vi "LimelightDistanceEstimator.vi"(1 "TargetHeight":dbl, 2 "Ty":dbl) -> (0 "Distance Estimate":dbl)   [LabVIEW 2018]
doc: "Takes in Target center pixel Y value (ty) and outputs the estimated distance of the target from the camera. This requires knowing the Angle the camera makes with the horizontal, camera height from ground, and target height from ground. Target height from ground is a required input."
panel:
  in  "CameraHeight":dbl
  in  "CameraAngle":dbl
  # "FIXED CAMERA ANGLE DISTANCE ESTIMATOR"
  # "This will be how far below the horizontal the camera views, since we've put it super high up and angled it down. \nPlease, just keep this number positive, in degrees"
  # "This is in inches. Measure from the floor, to the center of the lense."
  # "This is in inches. Measure from the floor, to the middle of the target (line connecting midpoints of angled tape inner edge)"
  # "Outputted Distance Estimate"
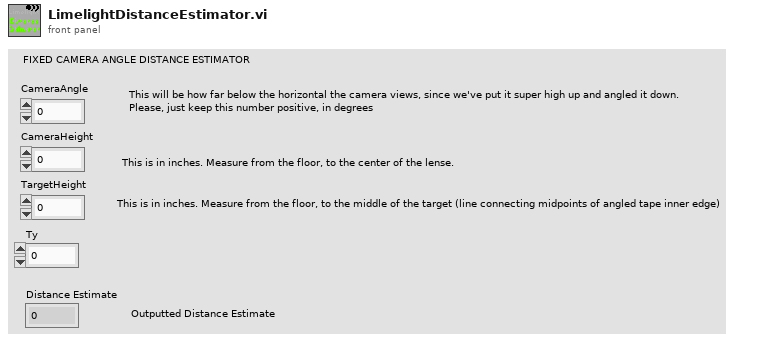
[diagram p1: front panel]
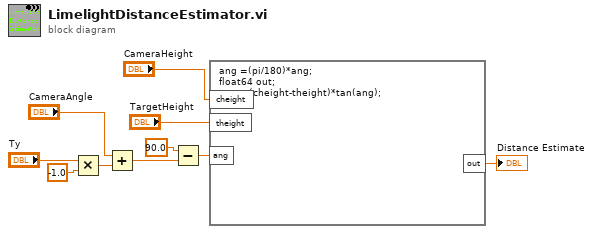
[diagram p0: block diagram]
diagram:
  n1 = Multiply(x="Ty", y=-1.0) -> (x*y=w3:dbl)
  n2 = Add(x="CameraAngle", y=w3) -> (x+y=w5:dbl)
  n3 = Subtract(x=90.0, y=w5) -> (x-y=w9:dbl)
  n4 = formula code="ang =(pi/180)*ang;\nfloat64 out;\nout = (cheight-theight)*tan(ang);"("cheight"="CameraHeight", "theight"="TargetHeight", "ang"=w9) -> ("out"=→"Distance Estimate":dbl)
